vi "DSO1K Edge Triggered Acquisition.vi"() -> ()   [LabVIEW 2009]
doc: "<B>This example shows how to configure the oscilloscope to perform an edge-triggered waveform acquisition.</B>"
uses:
  <instrlib>/DSO1K/Public/Data/Read Waveform (Single).vi
  <instrlib>/DSO1K/DSO1K.lvlib
panel:
  in  "Holdoff (4n)":dbl=4e-09 min=4e-09 max=10.0 format="%#_4p"
  in  "Trigger Mode (0:Auto)":u16(ring) items=["Auto (Untriggered Roll)", "Normal"]
  in  "Trigger Level (0V)":dbl min=-80.0 max=80.0 format="%#_4p"
  in  "Timebase (12:10us)":u16(ring)=12 items=["1ns", "2ns", "5ns", "10ns", "20ns", "50ns", "100ns", "200ns", "500ns", "1us", "2us", "5us", "10us", "20us", "50us", "100us", "200us", "500us", "1ms", "2ms", "5ms", "10ms", "20ms", "50ms", "100ms", "200ms", "500ms", "1s", "2s", "5s", "10s", "20s", "50s", "100s"]
  in  "Vertical Range (100m)":dbl=0.1 format="%#_4p"
  in  "Probe Attenuation (9:1X)":u16(ring)=9 items=["0.001 X", "0.002 X", "0.005 X", "0.01 X", "0.02 X", "0.05 X", "0.1 X", "0.2 X", "0.5 X", "1 X", "2 X", "5 X", "10 X", "20 X", "50 X", "100 X", "200 X", "500 X", "1k X"]
  in  "Vertical Coupling (0: DC)":u16(ring) items=["DC", "AC", "Ground"]
  in  "Channel (1: Channel 1)":u16(ring)=1 items=["Channel 1"=1, "Channel 2"=2, "Channel 3"=3, "Channel 4"=4]
  out "Waveform Graph":cluster{dbl, "Sampling Period":dbl, dbl[]}(graph)
  in  "VISA resource name":refnum<visa-resource-name>
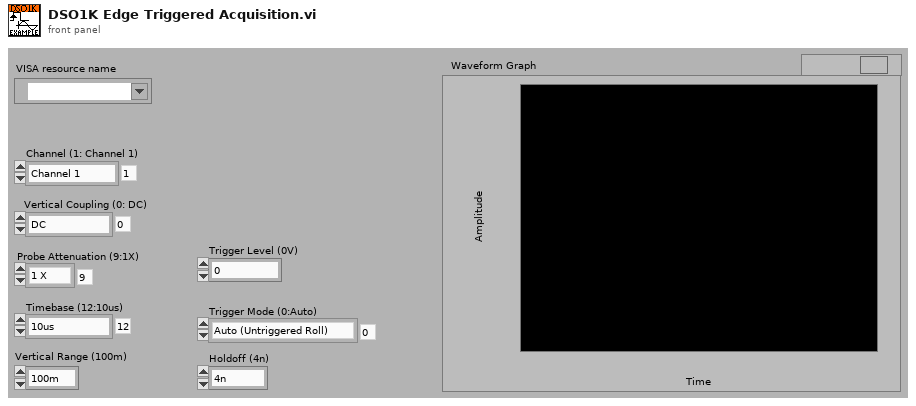
[diagram p1: front panel]
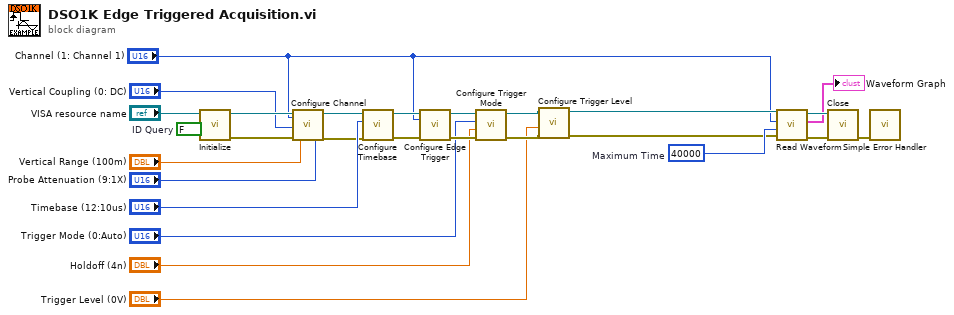
[diagram p0: block diagram]
diagram:
  w6 = FALSE  # ID Query
  w20 = u32 40000  # Maximum Time
  n1 = call <instrlib>:"Initialize.vi"("ID Query (True)"=w6, "VISA resource name"="VISA resource name") -> ("error out"=w24:errorcluster, "VISA resource name out"=w25:refnum<visa-resource-name>)  [unwired: 8 in]
  n2 = call <instrlib>:"Configure Channel.vi"("VISA resource name"=w25, "Channel (1: Channel 1)"="Channel (1: Channel 1)", "Vertical Coupling (0: DC)"="Vertical Coupling (0: DC)", "error in (no error)"=w24, "Vertical Range (100m)"="Vertical Range (100m)", "Probe Attenuation (9:1X)"="Probe Attenuation (9:1X)") -> ("VISA resource name out"=w3:refnum<visa-resource-name>, "error out"=w2:errorcluster)  [unwired: 12 in]
  n3 = call <instrlib>:"Configure Timebase.vi"("error in (no error)"=w2, "Timebase (12:10us)"="Timebase (12:10us)", "VISA resource name"=w3) -> ("error out"=w17:errorcluster, "VISA resource name out"=w18:refnum<visa-resource-name>)  [unwired: 7 in]
  n4 = call <instrlib>:"Configure Edge Trigger.vi"("VISA resource name"=w18, "Edge Trigger Source (1: Channel 1)"="Channel (1: Channel 1)", "error in (no error)"=w17) -> ("VISA resource name out"=w14:refnum<visa-resource-name>, "error out"=w15:errorcluster)  [unwired: 11 in]
  n5 = call <instrlib>:"Configure Trigger Mode.vi"("error in (no error)"=w15, "Holdoff (4n)"="Holdoff (4n)", "Trigger Mode (0:Auto)"="Trigger Mode (0:Auto)", "VISA resource name"=w14) -> ("error out"=w10:errorcluster, "VISA resource name out"=w11:refnum<visa-resource-name>)  [unwired: 6 in]
  n6 = call <instrlib>:"Configure Trigger Level.vi"("error in (no error)"=w10, "Trigger Level (0V)"="Trigger Level (0V)", "VISA resource name"=w11) -> ("error out"=w7:errorcluster, "VISA resource name out"=w8:refnum<visa-resource-name>)  [unwired: 7 in]
  n7 = call-poly <instrlib>:"Read Waveform.vi"("error in (no error)"=w7, "Timeout (40000 ms)"=w20, "Channel (1: Channel 1)"="Channel (1: Channel 1)", "VISA resource name"=w8) -> ("error out"=w21:errorcluster, "Waveform Graph"=→"Waveform Graph":cluster{dbl, "Sampling Period":dbl, dbl[]}, "VISA resource name out"=w23:refnum<visa-resource-name>)  [unwired: 4 in, 1 out]
  n8 = call <instrlib>:"Close.vi"("error in (no error)"=w21, "VISA resource name"=w23) -> ("error out"=w27:errorcluster)  [unwired: 9 in]
  n9 = call <vilib>:"Simple Error Handler.vi"("error in (no error)"=w27) -> ()  [unwired: 4 in, 5 out]
